vi "Create ByRef (DVR).vi"(8 "error in (no error)":errorcluster, 11 "Numeric in":refnum<class "Numeric Test Object.lvclass">) -> (0 "error out":errorcluster, 3 "Numeric out":refnum<class "Numeric Test Object.lvclass">)   [LabVIEW 2009, in "Numeric Test Object.lvclass"]
uses:
  Numeric Test Object.lvclass
  Numeric Test Object.lvclass/Numeric Test Object.ctl
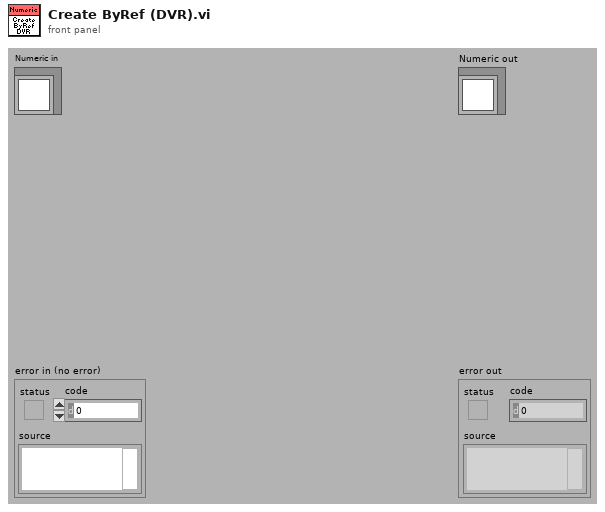
[diagram p1: front panel]
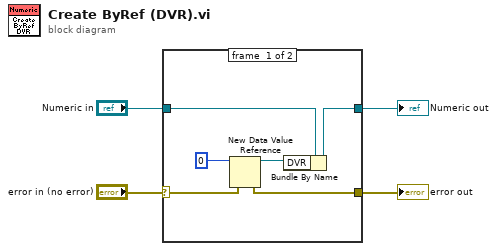
[diagram p0: block diagram]
diagram:
  n1 = case shown="No Error" "error in (no error)" {
    selector: "error in (no error)" -> [w6 w12]
    tunnel: [w5 w12] -> w3
    tunnel: [w9 w11] -> w1
    tunnel: "Numeric in" -> [w10 w11]
    frame #0 {
      n2 = New Data Value Reference(data value=0, error in=w6) -> (data value reference=w8:refnum<data-value>, error out=w5:errorcluster)
      n3 = Bundle By Name(cluster=w10, "DVR"=w8) -> (w9:refnum<class "Numeric Test Object.lvclass">)
    }
    frame #1 {
    }
  }
  "error out" <- w3
  "Numeric out" <- w1
